vi "Test Insert Tables without data2.vi"(11 "Test Case In":refnum<class "Test Open Xml.lvclass">) -> (0 "error out":errorcluster, 3 "Test Case Out":refnum<class "Test Open Xml.lvclass">)   [LabVIEW 2020, in "Test Open Xml.lvclass"]
uses:
  Test Open Xml.lvclass
  C:/Program Files/National Instruments/LabVIEW 2025/vi.lib/Astemes/LUnit/Test Case.lvclass
  <vilib>/Astemes/LUnit/Test Case.lvclass/Test Case.ctl
  Test Open Xml.lvclass/Test Open Xml.ctl
  Source/Open Xml.lvlib
  0a0d70f3-36fe-46ba-8b3e-e6c07e708d9f.vi
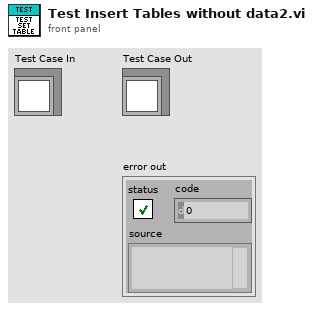
[diagram p1: front panel]
types:
  T1 = cluster{"Sheet Name":string, "Name":string, "Display Name":string, "Range or Cell Address":string}
  T2 = cluster{"Sheet Name":string, "Name":string, "Display Name":string, "Range":string}
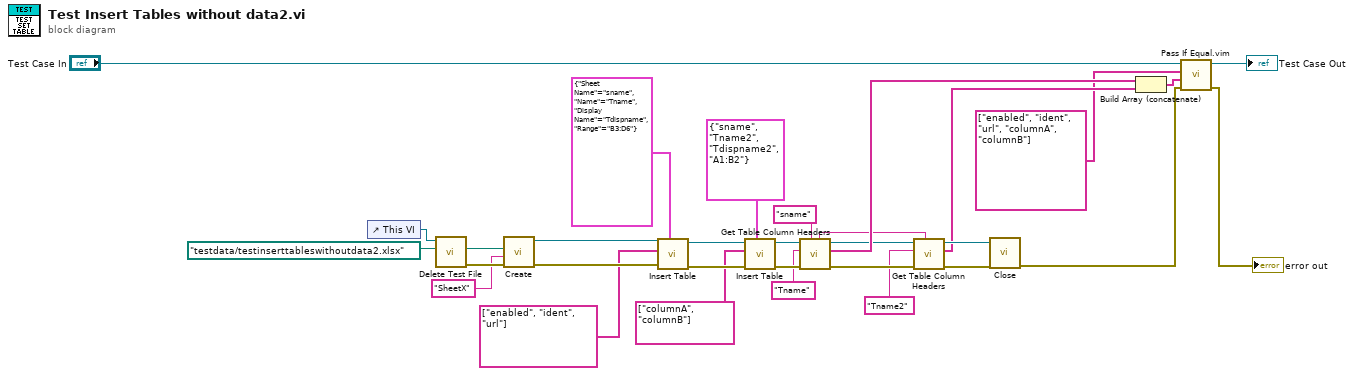
[diagram p0: block diagram]
diagram:
  n1 = control-ref of="This VI"() -> (w21:refnum<vi>)
  n2 = call "Delete Test File.vi"("name or relative path"=path "testdata/testinserttableswithoutdata2.xlsx", "VI in"=w21) -> ("error out"=w22:errorcluster, "deleted path"=w23:path)  [unwired: 8 in]
  n3 = call "Create.vi"("error in"=w22, "SheetName"="SheetX", "Path"=w23) -> ("error out"=w18:errorcluster, "SpreadsheetDoc"=w19:refnum<k24>)  [unwired: 7 in]
  n4 = call "Insert Table.vi"("Location"=T2 {"Sheet Name"="sname", "Name"="Tname", "Display Name"="Tdispname", "Range"="B3:D6"}, "error in"=w18, "Header Names"=string[] ["enabled", "ident", "url"], "SpreadsheetDoc in"=w19) -> ("error out"=w25:errorcluster, "SpreadsheetDoc out"=w14:refnum<k24>)  [unwired: 6 in]
  n5 = call "Insert Table.vi"("Location"=T1 {"Sheet Name"="sname", "Name"="Tname2", "Display Name"="Tdispname2", "Range or Cell Address"="A1:B2"}, "error in"=w25, "Header Names"=string[] ["columnA", "columnB"], "SpreadsheetDoc in"=w14) -> ("error out"=w15:errorcluster, "SpreadsheetDoc out"=w13:refnum<k24>)  [unwired: 6 in]
  n6 = call "Get Table Column Headers.vi"("Sheet Name in"="sname" ("Sheet Name"), "error in"=w15, "Table Name"="Tname", "SpreadsheetDoc in"=w13) -> ("error out"=w27:errorcluster, "Headers"=w26:string[], "SpreadsheetDoc out"=w9:refnum<k24>, "Sheet Name out"=w1:string)  [unwired: 4 in]
  n7 = call "Get Table Column Headers.vi"("Sheet Name in"=w1, "error in"=w27, "Table Name"="Tname2", "SpreadsheetDoc in"=w9) -> ("error out"=w10:errorcluster, "Headers"=w6:string[], "SpreadsheetDoc out"=w8:refnum<k24>)  [unwired: 4 in, 1 out]
  n8 = call "Close.vi"("error in"=w10, "SpreadsheetDoc"=w8) -> ("error out"=w28:errorcluster)  [unwired: 9 in]
  n9 = Build Array (concatenate)(w26, w6) -> (w7:string[])
  n10 = call "Pass If Equal.vim"("error in (no error)"=w28, "Actual"=w7, "Expected"=string[] ["enabled", "ident", "url", "columnA", "columnB"] ("Headers"), "LUnit Test Case In"="Test Case In") -> ("error out"=→"error out":errorcluster, "LUnit Test Case Out"=→"Test Case Out":refnum<class "Test Open Xml.lvclass">)  [unwired: 6 in]
